vi "Equip-Find Devices.vi"(7 "16-bit breakout":T1=enum."BNC-2090", 11 "error in (no error)":errorcluster) -> (4 "Num AO":i32[](array[numeric]), 6 "Num AI":i32[](array[numeric]), 8 "Slot Num":u32[](array[numeric]), 10 "connector types":T1[](array[typedef]), 14 "Trigger Slot":i32, 15 "error out":errorcluster)   [LabVIEW 2020]
uses:
  Type Defs/PXISlot XControl/Connector Type.ctl
  <resource>/objmgr/daqmx.rc
panel:
  out "Array":string[](array[string])
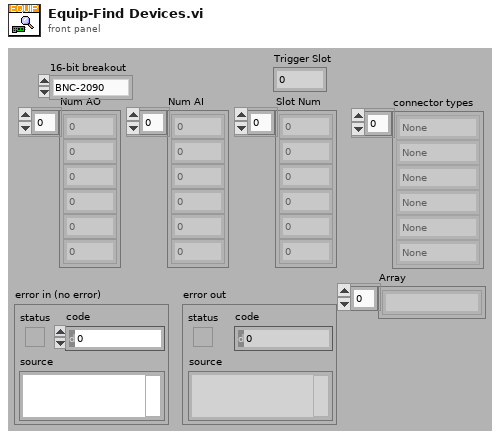
[diagram p1: front panel]
types:
  T1 = typedef "Connector Type.ctl" = enum16{"None", "PXI-4461", "BNC-2110", "BNC-2090", "PXIe-4463", "PXIe-4464"}
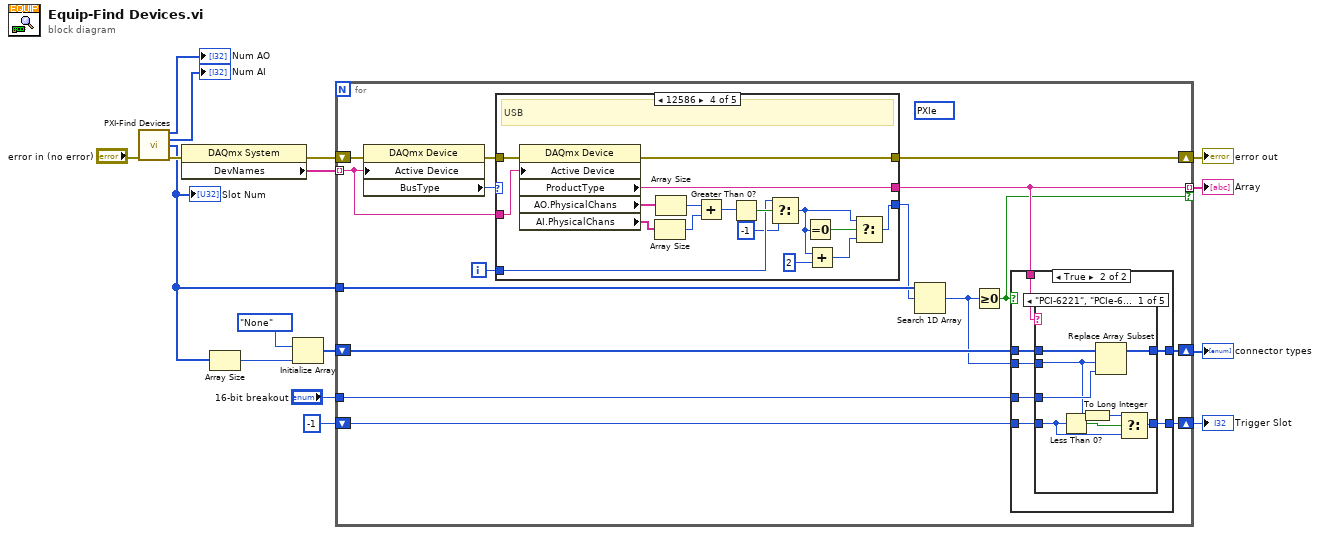
[diagram p0: block diagram]
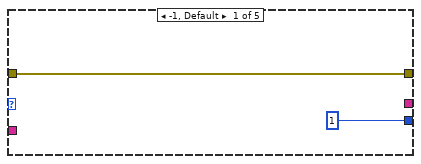
[diagram p2: hidden frame]
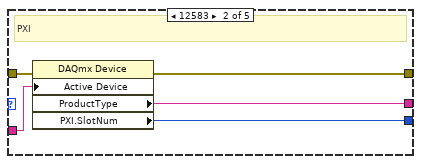
[diagram p3: hidden frame]
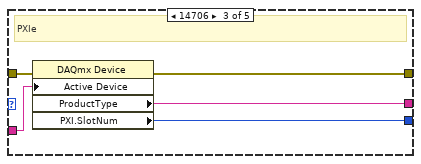
[diagram p4: hidden frame]
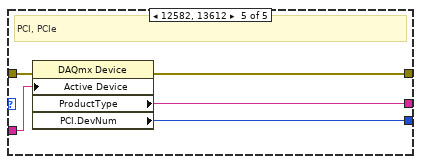
[diagram p5: hidden frame]
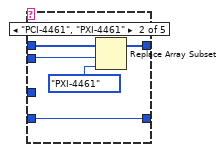
[diagram p7: hidden frame]
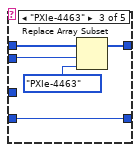
[diagram p8: hidden frame]
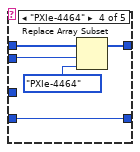
[diagram p9: hidden frame]
diagram:
  n1 = call "PXI-Find Devices.vi"("error in (no error)"="error in (no error)") -> ("Num AO"=→"Num AO":i32[], "Num AI"=→"Num AI":i32[], "Slot Num"=w3:u32[], "error out"=w10:errorcluster)  [unwired: 11 in]
  "Slot Num" <- w3
  n2 = property class="DAQmx System"(error in=w10) -> (error out=w15:errorcluster, "DevNames"=w16:tag[])  [unwired: 1 in, 1 out]
  n3 = Array Size(array=w3) -> (size(s)=w2:i32)
  n4 = Initialize Array(Connector_Type."None" ("Connector Type"), w2) -> (w12:T1[])
  n5 = for {
    tunnel: w16 -> [w21] mode=indexing
    shift-right: [w32] -> w14
    shift-left: w15 -> [w23]
    shift-right: [w30] -> w11
    shift-left: w12 -> [w31]
    tunnel: w3 -> [w29]
    tunnel: "16-bit breakout" -> [w27]
    shift-right: [w25] -> w4
    shift-left: -1 -> [w26]
    tunnel: [w19] -> w1 mode=indexing if=w17
    i -> [w20]
    (unwired) 14706 items=["PCI"=12582, "PCIe"=13612, "PXI"=12583, "PXIe"=14706, "SCXI"=12584, "SCC"=14707, "PCCard"=12585, "USB"=12586, "CompactDAQ"=14637, "TCP/IP"=14828, "Unknown"=12588, "SwitchBlock"=15870] ("BusType")
    n6 = property class="DAQmx Device"(error in=w23, "Active Device"=w21) -> (error out=w22:errorcluster, "BusType"=w18:i32)  [unwired: 1 in, 1 out]
    n7 = case shown="12586" w18 {
      tunnel: [_ w39 w44 w61 w66] -> w19
      tunnel: [w34 w38 w43 w60 w65] -> w32
      tunnel: [u32 1 ("PCI.DevNum") w37 w42 w48 w64] -> w28
      tunnel: w22 -> [w34 w36 w41 w59 w63]
      tunnel: w21 -> [_ w35 w40 w58 w62]
      tunnel: w20 -> [_ _ _ w51 _]
      frame -1, Default {
      }
      frame 12583 {
        # "PXI"
        n8 = property class="DAQmx Device"(error in=w36, "Active Device"=w35) -> (error out=w38:errorcluster, "ProductType"=w39:string, "PXI.SlotNum"=w37:u32)  [unwired: 1 in, 1 out]
      }
      frame 14706 {
        # "PXIe"
        n9 = property class="DAQmx Device"(error in=w41, "Active Device"=w40) -> (error out=w43:errorcluster, "ProductType"=w44:string, "PXI.SlotNum"=w42:u32)  [unwired: 1 in, 1 out]
      }
      frame 12586 {
        # "USB"
        n10 = property class="DAQmx Device"(error in=w59, "Active Device"=w58) -> (error out=w60:errorcluster, "ProductType"=w61:string, "AO.PhysicalChans"=w57:tag[], "AI.PhysicalChans"=w56:tag[])  [unwired: 1 in, 1 out]
        n11 = Array Size(array=w56) -> (size(s)=w54:i32)
        n12 = Array Size(array=w57) -> (size(s)=w55:i32)
        n13 = Add(x=w55, y=w54) -> (x+y=w53:i32)
        n14 = Greater Than 0?(x=w53) -> (x > 0?=w52:bool)
        n15 = Select(t=w51, s=w52, f=-1) -> (s? t:f=w47:i32)
        n16 = Equal To 0?(x=w47) -> (x = 0?=w49:bool)
        n17 = Add(x=w47, y=2) -> (x+y=w46:i32)
        n18 = Select(t=w47, s=w49, f=w46) -> (s? t:f=w48:i32)
      }
      frame 12582, 13612 {
        # "PCI, PCIe"
        n19 = property class="DAQmx Device"(error in=w63, "Active Device"=w62) -> (error out=w65:errorcluster, "ProductType"=w66:string, "PCI.DevNum"=w64:u32)  [unwired: 1 in, 1 out]
      }
    }
    n20 = Search 1D Array(1D array=w29, element=w28) -> (index of element=w24:i32)  [unwired: 1 in]
    n21 = Greater Or Equal To 0?(x=w24) -> (x >= 0?=w17:bool)
    n22 = case shown="True" w17 {
      tunnel: w19 -> [_ w75]
      tunnel: w31 -> [w68 w74]
      tunnel: [w68 w73] -> w30
      tunnel: w27 -> [_ w72]
      tunnel: w26 -> [w67 w71]
      tunnel: [w67 w70] -> w25
      tunnel: w24 -> [_ w69]
      frame False {
      }
      frame True {
        n23 = case shown="\"PCI-6221\", \"PCIe-6321\", \"PXI-6221\", \"PXIe-6341\", \"USB-6002\", \"USB-6221 (BNC)\", \"USB-6341 (BNC)\"" w75 {
          tunnel: w74 -> [w83 w88 w93 w98 w100]
          tunnel: [w82 w87 w92 w97 w100] -> w73
          tunnel: w69 -> [w78 w85 w90 w95 _]
          tunnel: w72 -> [w81 _ _ _ _]
          tunnel: w71 -> [w77 w84 w89 w94 w99]
          tunnel: [w80 w84 w89 w94 w99] -> w70
          frame "PCI-6221", "PCIe-6321", "PXI-6221", "PXIe-6341", "USB-6002", "USB-6221 (BNC)", "USB-6341 (BNC)" {
            n24 = Less Than 0?(x=w77) -> (x < 0?=w79:bool)
            n25 = To Long Integer(number=w78) -> (32bit integer=w76:i32)
            n26 = Replace Array Subset(array=w83, new element=w81, index=w78) -> (w82:T1[])
            n27 = Select(t=w76, s=w79, f=w77) -> (s? t:f=w80:i32)
          }
          frame "PCI-4461", "PXI-4461" {
            n28 = Replace Array Subset(array=w88, new element=Connector_Type."PXI-4461" ("Connector Type"), index=w85) -> (w87:T1[])
          }
          frame "PXIe-4463" {
            n29 = Replace Array Subset(array=w93, new element=Connector_Type."PXIe-4463" ("Connector Type"), index=w90) -> (w92:T1[])
          }
          frame "PXIe-4464" {
            n30 = Replace Array Subset(array=w98, new element=Connector_Type."PXIe-4464" ("Connector Type"), index=w95) -> (w97:T1[])
          }
          frame "", Default {
          }
        }
      }
    }
  }
  "error out" <- w14
  "connector types" <- w11
  "Trigger Slot" <- w4
  "Array" <- w1
